vi "Multiplier1.vi"() -> (8 "Multiplier1":refnum<class "Multiplier1.lvclass">)   [LabVIEW 2017, in "Multiplier1.lvclass"]
uses:
  Multiplier1.lvclass
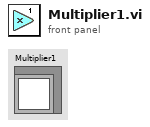
[diagram p1: front panel]
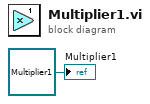
[diagram p0: block diagram]
diagram:
  "Multiplier1" <- refnum<class "Multiplier1.lvclass"> refnum ("Multiplier1.lvclass")
